vi "Make random GB Script.vi"() -> ()   [LabVIEW 2010]
panel:
  out "# of Reduced":i32
  in  "Relaxation Type":string(combo)="conv opti"
  out "Subset for Y?":bool=TRUE
  out "Subset for X?":bool
  out "Index":i32
  in  "Reduce to Repeating":T1={"Slab X"=4.6, "Slab Y"=4.0, "Tolerance (A)"=0.5, "Presorted?"=FALSE}
  in  "Grain Growth and Geometry":T2={"Grain 1 Length (A)"=23.0, "Grain 2 Length (A)"=23.0, "Max Grain Height"=80.0, "Max Grain Width"=14.01, "Grain 1 Start"=0.0, "Overlap Region (A)"=0.0}
  in  "Path":path
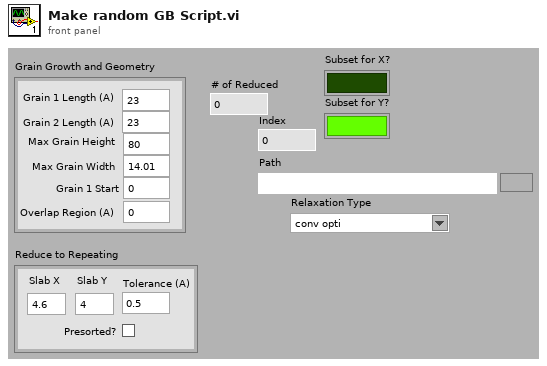
[diagram p1: front panel]
types:
  T1 = cluster{"Slab X":dbl, "Slab Y":dbl, "Tolerance (A)":dbl, "Presorted?":bool}
  T2 = cluster{"Grain 1 Length (A)":dbl, "Grain 2 Length (A)":dbl, "Max Grain Height":dbl, "Max Grain Width":dbl, "Grain 1 Start":dbl, "Overlap Region (A)":dbl}
  T3 = cluster{"Grain 1 Orientation":dbl[], "Grain 2 Orientation":dbl[], "Twist Angle (Deg)":dbl, "Translation Vector":dbl[]}
  T4 = cluster{"Structure Name":string, "Lattice vector a":dbl[], "Lattice vector b":dbl[], "Lattice vector c":dbl[], "Atoms Array":cluster{"Atom Name":string, "Positions (Direct)":dbl[][], "Positions (Cartesian)":dbl[][]}[], "# of atoms":i32}
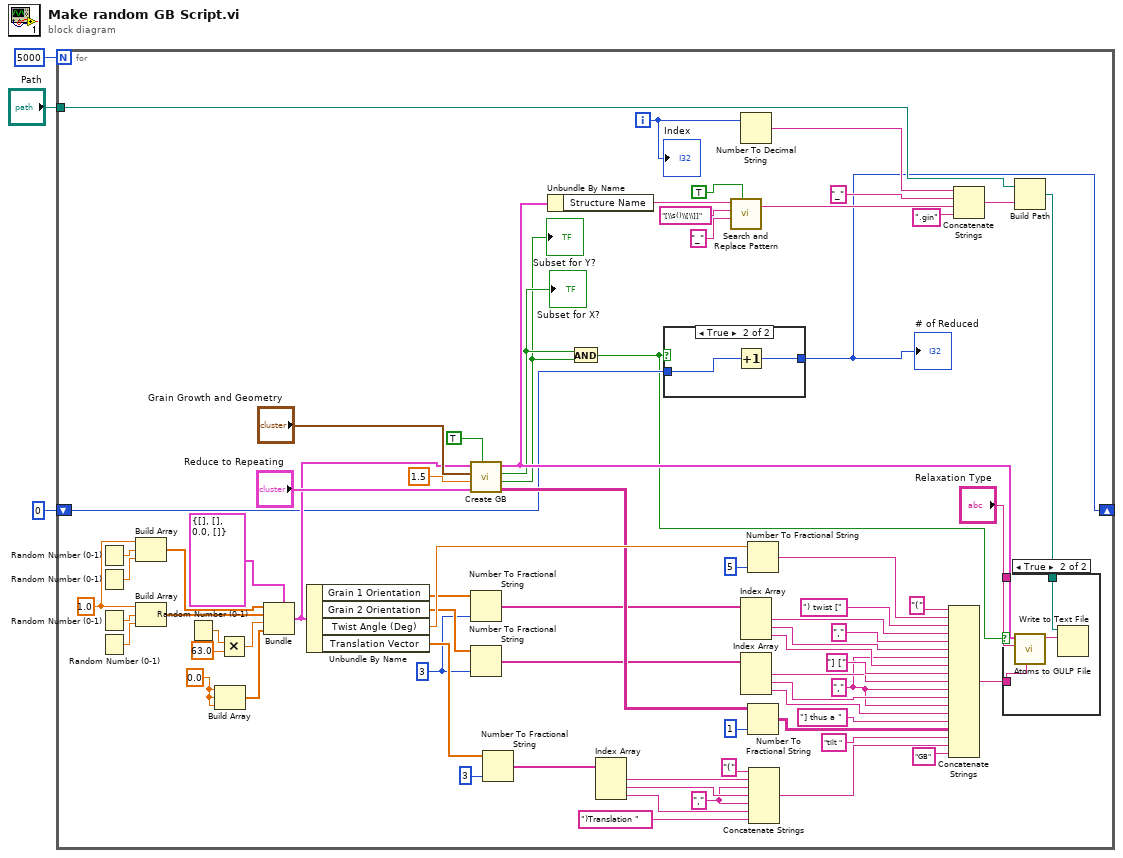
[diagram p0: block diagram]
diagram:
  n1 = for {
    N: 5000 -> [_]
    tunnel: "Path" -> [w59]
    shift-right: [w6] -> _
    shift-left: 0 -> [w7]
    i -> [w63]
    w17 = i16 3 ("precision (6)")
    w31 = "," ("string")
    w42 = "," ("string")
    w66 = 0.0 ("element")
    w74 = 1.0
    n2 = Random Number (0-1)() -> (number: 0 to 1=w76:dbl)
    n3 = Random Number (0-1)() -> (number: 0 to 1=w75:dbl)
    n4 = Random Number (0-1)() -> (number: 0 to 1=w73:dbl)
    n5 = Random Number (0-1)() -> (number: 0 to 1=w72:dbl)
    n6 = Build Array(w74, w76, w75) -> (w71:dbl[])
    n7 = Build Array(w74, w73, w72) -> (w70:dbl[])
    n8 = Random Number (0-1)() -> (number: 0 to 1=w69:dbl)
    n9 = Build Array(w66, w66, w66) -> (w65:dbl[])
    n10 = Multiply(x=w69, y=63.0) -> (x*y=w67:dbl)
    n11 = Bundle(cluster=T3 {"Grain 1 Orientation"=[], "Grain 2 Orientation"=[], "Twist Angle (Deg)"=0.0, "Translation Vector"=[]} ("Grain Boundary Definition"), "Grain 1 Orientation"=w71, "Grain 2 Orientation"=w70, "Twist Angle (Deg)"=w67, "Translation Vector"=w65) -> (w22:T3)
    n12 = Unbundle By Name(w22) -> ("Grain 1 Orientation"=w21:dbl[], "Grain 2 Orientation"=w19:dbl[], "Twist Angle (Deg)"=w26:dbl, "Translation Vector"=w25:dbl[])
    n13 = call "Create GB.vi"("Skip cleanup if no subset"=TRUE ("Skip crop if no subset"), "Reduce to Repeating"="Reduce to Repeating", "Min Seperation Distance (A)"=1.5, "Grain Growth and Geometry"="Grain Growth and Geometry", "Grain Boundary Definition"=w22) -> ("GB Data"=w24:string[][], "Reduced Orthorhombic?"=w8:bool, "Reduced Rhombahedral?"=w9:bool, "Grain Boundary"=w64:T4)  [unwired: 2 in, 1 out]
    "Subset for X?" <- w9
    "Subset for Y?" <- w8
    n14 = Number To Fractional String(number=w21, precision (6)=w17) -> (F-format string=w20:string[])  [unwired: 2 in]
    n15 = Number To Fractional String(number=w19, precision (6)=w17) -> (F-format string=w18:string[])  [unwired: 2 in]
    n16 = Number To Fractional String(number=w25, precision (6)=i16 3) -> (F-format string=w35:string[])  [unwired: 2 in]
    n17 = Unbundle By Name(w64) -> ("Structure Name"=w12:string)
    n18 = And(x=w9, y=w8) -> (x .and. y?=w5:bool)
    n19 = Index Array(array=w35) -> (element #1=w34:string, element #2=w32:string, element #3=w30:string)  [unwired: 3 in]
    n20 = case shown="True" w5 {
      tunnel: w7 -> [w82 w84]
      tunnel: [w82 w83] -> w6
      frame False {
      }
      frame True {
        n21 = Increment(x=w84) -> (x+1=w83:i32)
      }
    }
    "# of Reduced" <- w6
    n22 = call <vilib>:"Search and Replace Pattern.vi"("string"=w12, "regular expression (\"\")"="[\\s()\\[\\]]" ("regular expression (\"\")"), "replace string (\"\")"="_" ("replace string (\"\")"), "replace all? (F)"=TRUE) -> ("result string"=w11:string)  [unwired: 1 in, 1 out]
    n23 = Number To Decimal String(number=w63) -> (decimal integer string=w62:string)  [unwired: 1 in]
    n24 = Index Array(array=w20) -> (element #1=w49:string, element #2=w47:string, element #3=w46:string)  [unwired: 3 in]
    n25 = Index Array(array=w18) -> (element #1=w44:string, element #2=w43:string, element #3=w41:string)  [unwired: 3 in]
    n26 = Number To Fractional String(number=w26, precision (6)=i16 5) -> (F-format string=w51:string)  [unwired: 2 in]
    n27 = Number To Fractional String(number=w24, precision (6)=i16 1) -> (F-format string=w39:string[][])  [unwired: 2 in]
    n28 = Concatenate Strings("(" ("string"), w34, w31, w32, w31, w30, ")Translation " ("string")) -> (w28:string)
    n29 = Concatenate Strings("(" ("string"), w51, ") twist [" ("string"), w49, "," ("string"), w47, w42, w46, "] [" ("string"), w44, w42, w43, w42, w41, "] thus a " ("string"), w39, "tilt " ("string"), w28, "GB" ("string")) -> (w16:string)
    n30 = Concatenate Strings(w62, "_" ("string"), w11, ".gin" ("string")) -> (w61:string)
    n31 = Build Path(base path=w59, name or relative path=w61) -> (appended path=w60:path)
    n32 = case shown="True" w5 {
      tunnel: w64 -> [_ w80]
      tunnel: w60 -> [_ w79]
      tunnel: w16 -> [_ w78]
      tunnel: "Relaxation Type" -> [_ w77]
      frame False {
      }
      frame True {
        n33 = call "Atoms to GULP File.vi"("Potentials"=w78, "Relaxation Type"=w77, "Structure"=w80) -> ("GULP File"=w81:string)  [unwired: 8 in]
        n34 = Write to Text File(file (use dialog)=w79, text=w81) -> ()  [unwired: 2 in, 3 out]
      }
    }
    "Index" <- w63
  }
